vi "Run_Expand_Z_Object_decomposition.vi"() -> (0 "object cluster":T1)   [LabVIEW 2019]
uses:
  <vilib>/Utility/file.llb/Read Delimited Spreadsheet (DBL).vi
panel:
  out "Omega":dbl[][](array[numeric])
  out "object":dbl[](array[numeric])
  in  "Lq":i32=15
  out "OmegaChain":dbl[](array[numeric])
  out "beta":dbl[](array[numeric])
  out "gamma":dbl
  out "weight":dbl
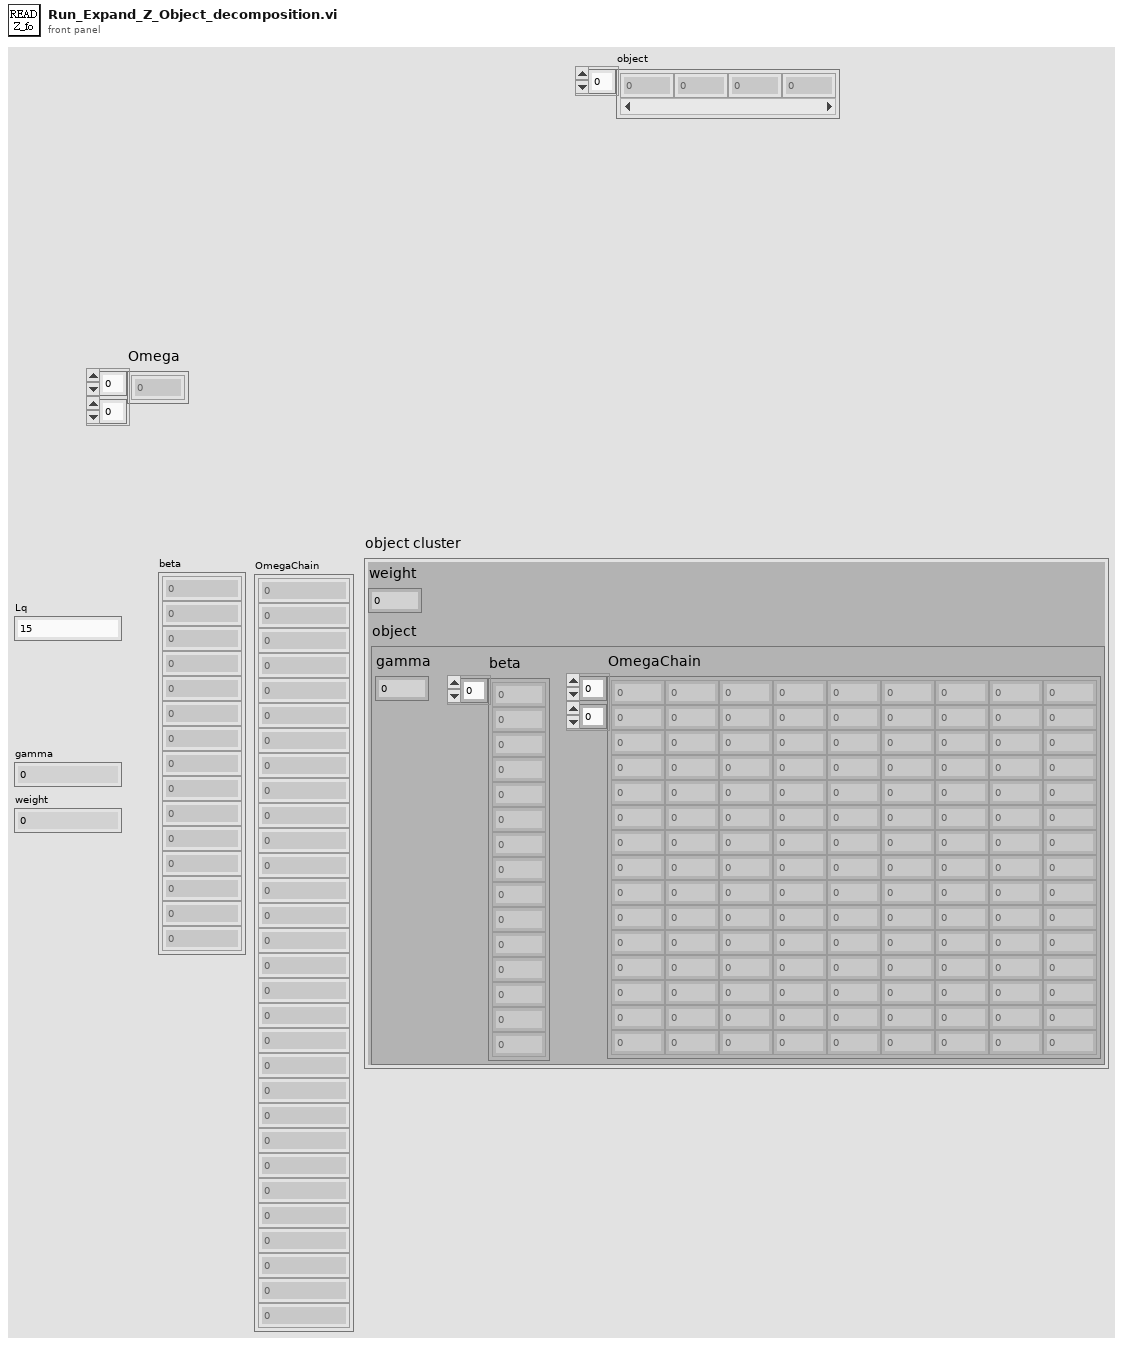
[diagram p1: front panel]
types:
  T1 = cluster{"weight":dbl, "object":cluster{"beta":dbl[], "gamma":dbl, "OmegaChain":dbl[][]}}
  T2 = cluster{"beta":dbl[], "gamma":dbl, "OmegaChain":dbl[][]}
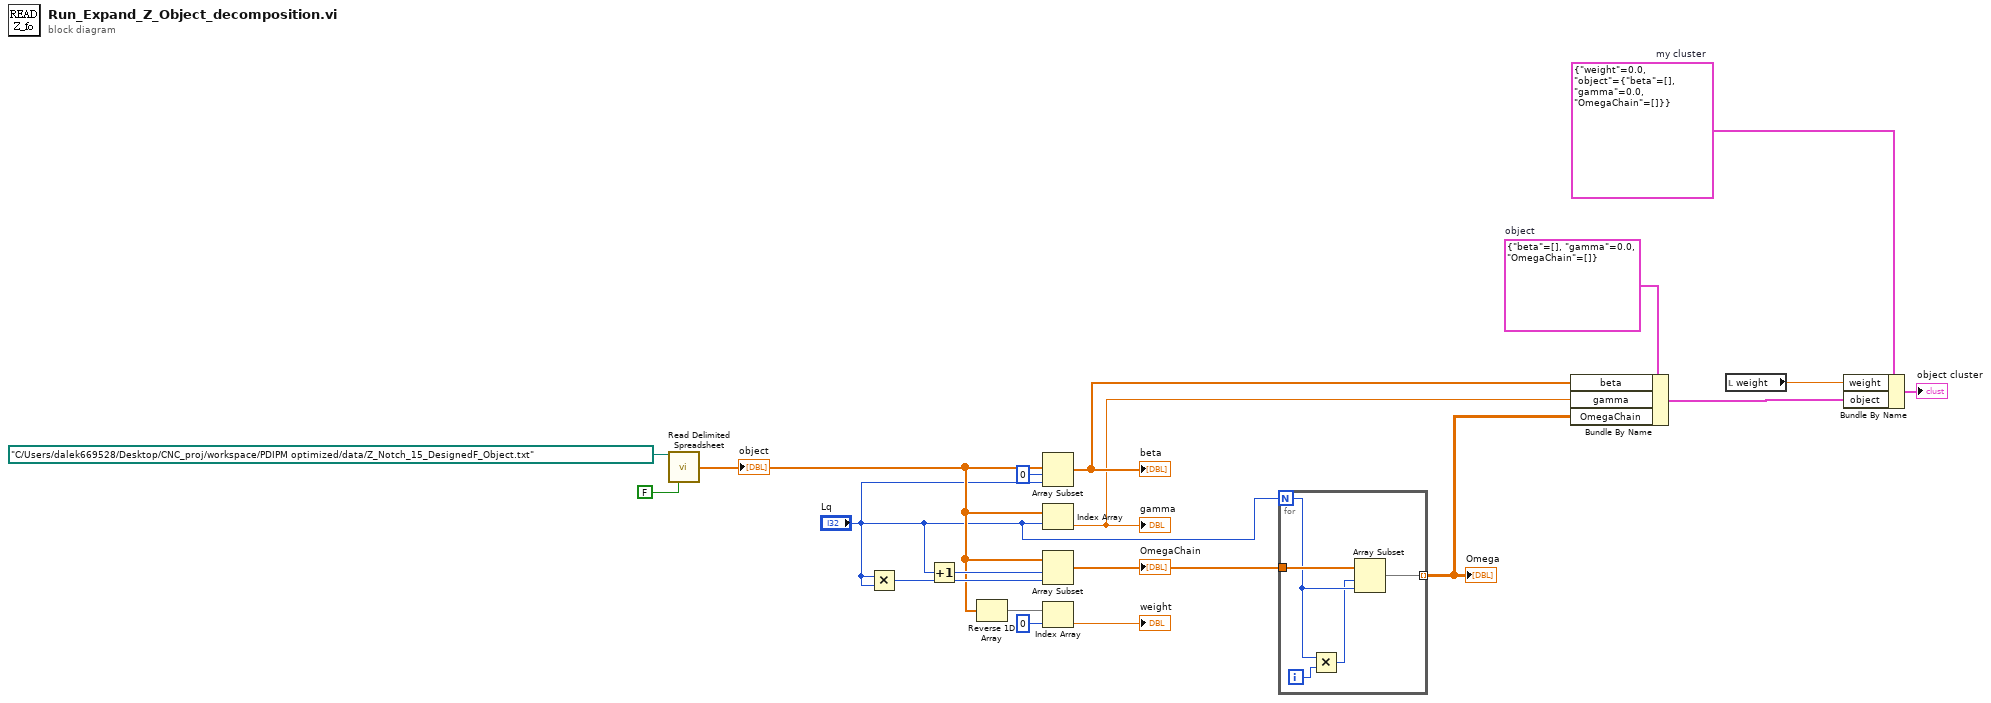
[diagram p0: block diagram]
diagram:
  w6 = T2 {"beta"=[], "gamma"=0.0, "OmegaChain"=[]}  # object
  w7 = T1 {"weight"=0.0, "object"={"beta"=[], "gamma"=0.0, "OmegaChain"=[]}}  # my cluster
  n1 = call-poly <vilib>:"Read Delimited Spreadsheet.vi"("file path (dialog if empty)"=path "C:/Users/dalek669528/Desktop/CNC_proj/workspace/PDIPM optimized/data/Z_Notch_15_DesignedF_Object.txt", "transpose? (F)"=FALSE) -> ("first row"=w9:dbl[])  [unwired: 8 in, 5 out]
  "object" <- w9
  n2 = Multiply(x="Lq", y="Lq") -> (x*y=w10:i32)
  n3 = Increment(x="Lq") -> (x+1=w16:i32)
  n4 = Reverse 1D Array(array=w9) -> (reversed array=w15:dbl[])
  n5 = Array Subset(array=w9, index=0, length="Lq") -> (w13:dbl[])
  "beta" <- w13
  n6 = Index Array(array=w9, index="Lq") -> (element=w12:dbl)
  "gamma" <- w12
  n7 = Array Subset(array=w9, index=w16, length=w10) -> (w3:dbl[])
  "OmegaChain" <- w3
  n8 = Index Array(array=w15, index=0) -> (element=→"weight":dbl)
  n9 = for {
    N: "Lq" -> [w22]
    tunnel: w3 -> [w24]
    tunnel: [w20] -> w2 mode=indexing
    i -> [w23]
    n10 = Multiply(x=w22, y=w23) -> (x*y=w21:i32)
    n11 = Array Subset(array=w24, index=w21, length=w22) -> (w20:dbl[])
  }
  "Omega" <- w2
  n12 = Bundle By Name(cluster=w6, "beta"=w13, "gamma"=w12, "OmegaChain"=w2) -> (w5:T2)
  n13 = local read "weight"() -> (w8:dbl)
  n14 = Bundle By Name(cluster=w7, "weight"=w8, "object"=w5) -> (→"object cluster":T1)
